vi "UT_FileHandler_Main.vi"(8 "error in":errorcluster) -> (0 "error out":errorcluster)   [LabVIEW 2016, in "UT_FileHandler.lvlib"]
doc: "Collection of tests for the FileHandler class."
uses:
  UT_FileHandler.lvlib
  <vilib>/addons/_JKI Toolkits/Caraya/classes/Test/Test.lvclass
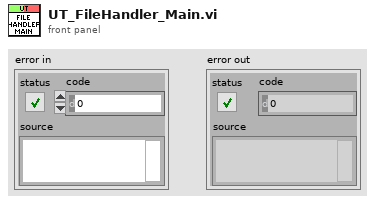
[diagram p1: front panel]
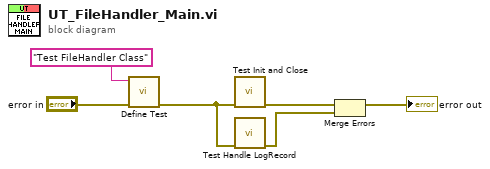
[diagram p0: block diagram]
diagram:
  n1 = call <vilib>:"Define Test.vi"("error in (no error)"="error in", "Label (VI Title)"="Test FileHandler Class") -> ("error out"=w5:errorcluster)  [unwired: 8 in, 1 out]
  n2 = call "Test Init and Close.vi"("error in"=w5) -> ("error out"=w4:errorcluster)  [unwired: 10 in]
  n3 = call "Test Handle LogRecord.vi"("error in"=w5) -> ("error out"=w3:errorcluster)  [unwired: 10 in]
  n4 = Merge Errors(w4, w3) -> (→"error out":errorcluster)
